vi "In_S10F3.vi"(8 "error in (no error)":errorcluster, 11 "S10 Message Class in":refnum<class "S10 Message Class.lvclass">) -> (0 "error out":errorcluster, 1 "OK?":bool, 2 "S10F3":T1, 3 "S10 Message Class out":refnum<class "S10 Message Class.lvclass">)   [LabVIEW 2020, in "SECS Communication.lvlib" / "S10 Message Class.lvclass"]
uses:
  S10 Message Class.lvclass
  D:/Dropbox/SECS/SECS_GEM v1.0.6/Com/SECS Communication/SECS-II Class/SECS-II Class.lvclass
  S10F3.ctl
  SECS-II Class/SECS-II Class.lvclass/SECS-II Class.ctl
  SECS-II Class/Variant To Data_Binary.vi
  SECS-II Class/Variant To Data_ASCII.vi
  SECS-II Class/SECS-II Class.lvclass
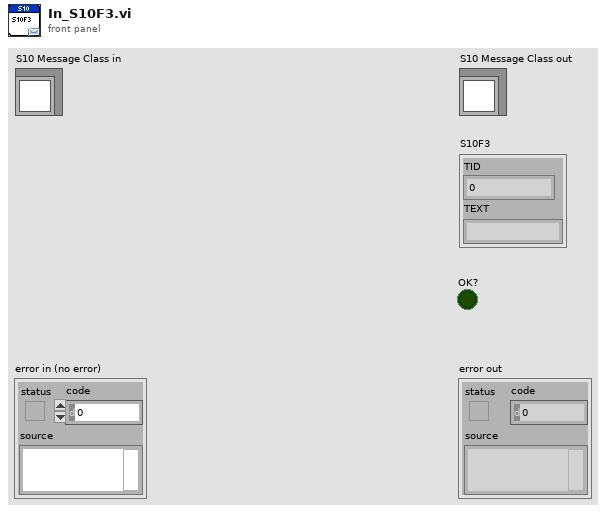
[diagram p1: front panel]
types:
  T1 = typedef "SECS Communication.lvlib/S10 Message Class.lvclass/S10F3.ctl" = cluster{"TID":u8, "TEXT":string}
  T2 = typedef "SECS Communication.lvlib/SECS-II Class.lvclass/Message Data.ctl" = cluster{"Index":i32, "Data Item Format":T3, "Format Code":T4, "Parent Index":i32, "Child Index":i32[], "Data":variant}
  T3 = typedef "SECS Communication.lvlib/SECS-II Class.lvclass/Data Item Format.ctl" = enum16{"Data Type", "Value"}
  T4 = typedef "SECS Communication.lvlib/SECS-II Class.lvclass/Format Code.ctl" = enum16{"L", "A", "B", "Boolean", "J", "I1", "I2", "I4", "I8", "U1", "U2", "U4", "U8", "F4", "F8", "Char"}
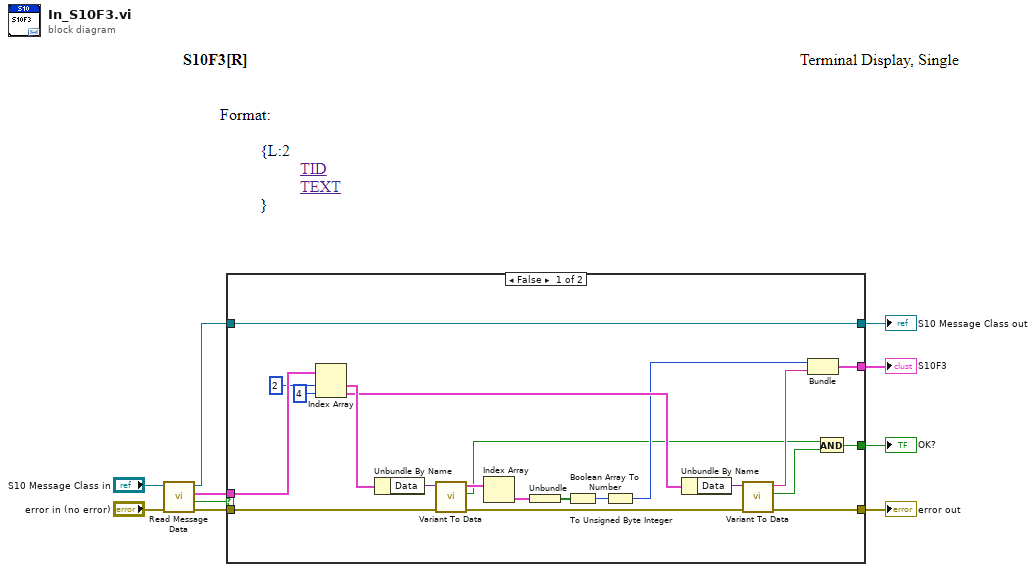
[diagram p0: block diagram]
diagram:
  n1 = call "Read Message Data.vi"("error in (no error)"="error in (no error)", "SECS-II Class in"="S10 Message Class in") -> ("error out"=w10:errorcluster, "Empty?"=w3:bool, "Message Data"=w9:T2[], "SECS-II Class out"=w1:refnum<class "S10 Message Class.lvclass">)  [unwired: 6 in]
  n2 = case shown="False" w3 {
    tunnel: w10 -> [w31 w33]
    tunnel: w9 -> [w30 _]
    tunnel: [w22 w33] -> w8
    tunnel: [w21 _] -> w7
    tunnel: [w12 _] -> w4
    tunnel: [w11 w32] -> w2
    tunnel: w1 -> [w11 w32]
    frame False {
      n3 = Index Array(array=w30, index #1=2 ("index"), index #2=4 ("index")) -> (element #1=w26:T2, element #2=w25:T2)
      n4 = Unbundle By Name(w26) -> ("Data"=w29:variant)
      n5 = call-poly "Variant To Data.vi"("error in (no error)"=w31, "Variant"=w29) -> ("error out"=w24:errorcluster, "OK?"=w13:bool, "Data Cluster"=w19:cluster{"Data":bool[]}[])  [unwired: 7 in]
      n6 = Index Array(array=w19) -> (element=w18:cluster{"Data":bool[]})  [unwired: 1 in]
      n7 = Unbundle(w18) -> ("Data"=w17:bool[])
      n8 = Boolean Array To Number(Boolean array=w17) -> (number=w16:u32)
      n9 = To Unsigned Byte Integer(number=w16) -> (unsigned 8bit integer=w15:u8)
      n10 = Unbundle By Name(w25) -> ("Data"=w23:variant)
      n11 = call-poly "Variant To Data.vi"("error in (no error)"=w24, "Variant"=w23) -> ("error out"=w22:errorcluster, "OK?"=w14:bool, "Data"=w20:string)  [unwired: 7 in]
      n12 = Bundle(w15, "Data"=w20) -> (w21:cluster{u8, "Data":string})  [unwired: 1 in]
      n13 = And(x=w13, y=w14) -> (x .and. y?=w12:bool)
    }
    frame True {
    }
  }
  "error out" <- w8
  "S10 Message Class out" <- w2
  "S10F3" <- w7
  "OK?" <- w4
